vi "Autonomous Independent.vi"() -> ()   [LabVIEW 2016]
doc: "This VI is called when autonomous begins, and will automatically be terminated when autonomous ends. You can carry out timed or sensor driven robot movement independently without needing to return to the caller."
uses:
  <vilib>/Rock Robotics/WPI/ThirdParty/CanMotor/TalonSRX/WPI_CANTalonSRX_APIFeedbackSelect.ctl
  <vilib>/Rock Robotics/WPI/ThirdParty/CanMotor/TalonSRX/WPI_CANTalonSRX_Params.ctl
  <vilib>/Rock Robotics/WPI/ThirdParty/CanMotor/TalonSRX/WPI_CANTalonSRX_APIControlMode.ctl
  <vilib>/Rock Robotics/WPI/Utilities/WPI_GetSetVariantRefNum.vi
  <vilib>/Rock Robotics/Network Tables/NT Read String.vi
  <vilib>/Rock Robotics/Network Tables/NT Write Numeric Array.vi
  <vilib>/Rock Robotics/WPI/RobotDrive/WPI_RobotDriveArcadeDrive_Standard(NoSaturation).vi
  Robot Global Data.vi
panel:
  out "RIGHT SIDE":dbl
  out "Encoder Position 4":dbl
  out "Encoder Position 3":dbl
  out "Encoder Position":dbl
  out "Encoder Position 2":dbl
  # "Be sure to right-click and choose Data Operations>>Make Current Value default if you want to save the array values with the VI"
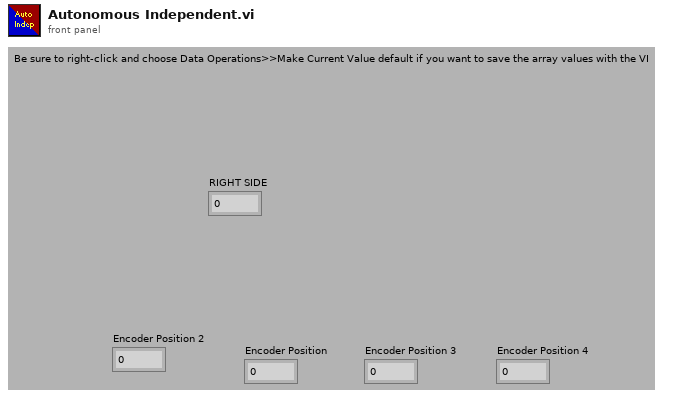
[diagram p1: front panel]
types:
  T1 = typedef "WPI_JoystickDevRef.ctl" = cluster{"Device":T2}
  T2 = typedef "WPI_JoystickDeviceEnum.ctl" = enum16{"USB 0", "USB 1", "USB 2", "USB 3", "USB 4", "USB 5"}
  T3 = typedef "WPI_EncoderDevRef.ctl" = cluster{"DevStatus":errorcluster, "EncoderIndex":T4, "CounterIndex":T5, "DistancePerCount":dbl, "Decoding Type":T6}
  T4 = typedef "FPGA_EncoderIdx.ctl" = enum8{"Enc 0", "Enc 1", "Enc 2", "Enc 3", "Enc 4", "Enc 5", "Enc 6", "Enc 7", "Invalid"}
  T5 = typedef "FPGA_CounterCtrSystemIndex.ctl" = enum8{"Ctr 0", "Ctr 1", "Ctr 2", "Ctr 3", "Ctr 4", "Ctr 5", "Ctr 6", "Ctr 7", "Invalid"}
  T6 = typedef "WPI_EncoderType.ctl" = enum16{"1x", "2x", "4x"}
  T7 = typedef "WPI_MotorControlDeviceRef.ctl" = cluster{"DeviceStatus":errorcluster, "Type":T8, "PWM":cluster{"PWM Channel":T9, "DeadBand":T10}, "CAN":cluster{"Device Number":u8, "SetOutput VI Ref":variant, "GetOutput VI Ref":variant, "Enable VI Ref":variant, "Disable VI Ref":variant, "Data":variant}, "Invert":bool}
  T8 = typedef "WPI_MotorControlType.ctl" = enum16{"PWM", "CAN"}
  T9 = typedef "FPGA_DIOPWMChannel.ctl" = enum8{"PWM 0", "PWM 1", "PWM 2", "PWM 3", "PWM 4", "PWM 5", "PWM 6", "PWM 7", "PWM 8", "PWM 9", "PWM MXP 0", "PWM MXP 1", "PWM MXP 2", "PWM MXP 3", "PWM MXP 4", "PWM MXP 5", "PWM MXP 6", "PWM MXP 7", "PWM MXP 8", "PWM MXP 9", "Invalid"}
  T10 = typedef "WPI_PWMDeadband.ctl" = cluster{"Name":string, "maxPositivePwm":i32, "minPositivePwm":i32, "centerPwm":i32, "maxNegativePwm":i32, "minNegativePwm":i32, "angularRange":u16}
  T11 = typedef "WPI_RobotDriveDevRef.ctl" = cluster{"DevStatus":errorcluster, "Motors[]":T7[], "Square Inputs":bool, "Max Output":dbl}
  T12 = typedef "WPI_CANTalonSRX_APIFeedbackSelect.ctl" = enum16{"Digital Quadrature Encoder", "Analog Potentiometer", "Analog Encoder", "Count on Quad-A (Rising-Edge)", "Count on Quad-A (Falling-Edge)", "CTR Magnetic Enc (Absolute)", "CTR Magnetic Enc (Relative)", "Pulse Width"}
  T13 = typedef "WPI_CANTalonSRX_APIControlMode.ctl" = enum8{"Percent VBus", "Speed", "Position", "Slave", "Unchanged / Invalid", "Voltage Compensation", "Current", "Motion Profile", "Motion Magic"}
  T14 = typedef "WPI_CANTalonSRX_Params.ctl" = u8
  T15 = typedef "WPI_CANTalonSRX_GlobalStatus.ctl" = cluster{"Applied Throttle":dbl, "Module Enabled":bool, "CAN Error":errorcluster, "Closed Loop Error":dbl, "Forward Limit Switch Closed":bool, "Reverse Limit Switch Closed":bool, "Sensor Position":dbl, "Sensor Velocity":dbl, "Current":dbl, "Sticky Fault - Over Temp":bool, "Sticky Fault - Under Voltage":bool, "Sticky Fault - Forward Limit":bool, "Sticky Fault - Reverse Limit":bool, "Sticky Fault - Forward Soft Limit":bool, "Sticky Fault - Reverse Soft Limit":bool, "Brake is Enabled":bool, "Encoder Position":dbl, "Encoder Velocity":dbl, "Encoder Index Count":dbl, "Encoder A Pin State":bool, "Encoder B Pin State":bool, "Encoder Index Pin State":bool, "Analog In":dbl, "Analog In Velocity":dbl, "Temperature (C)":dbl, "Battery Voltage":dbl, "Control 5 Is Supported":bool, "Current Profile Slot Select":dbl, "Pos Div 8":bool, "Vel Div 4":bool, "Pulse Width Position":i32, "Pulse Width Velocity":i32, "Pulse Width Rise To Rise (us)":i32, "Pulse Width Rise To Fall (us)":i32, "Mot Prof Active Is Under Run":bool, "Mot Prof Active Has Under Run":bool, "Mot Prof Active Is Last":bool, "Mot Prof Active Velocity Only":bool, "Mot Prof Active Is Valid":bool, "Mot Prof Buffer Is Full":bool, "Mot Prof Active Profile Slot Select":i32, "Mot Prof NextID":i32, "Mot Prof Count":i32, "Mot Prof Active Velocity":dbl, "Mot Prof Active Position":dbl, "Mot Prof Output Enable":i32, "UsageFrame":u32}
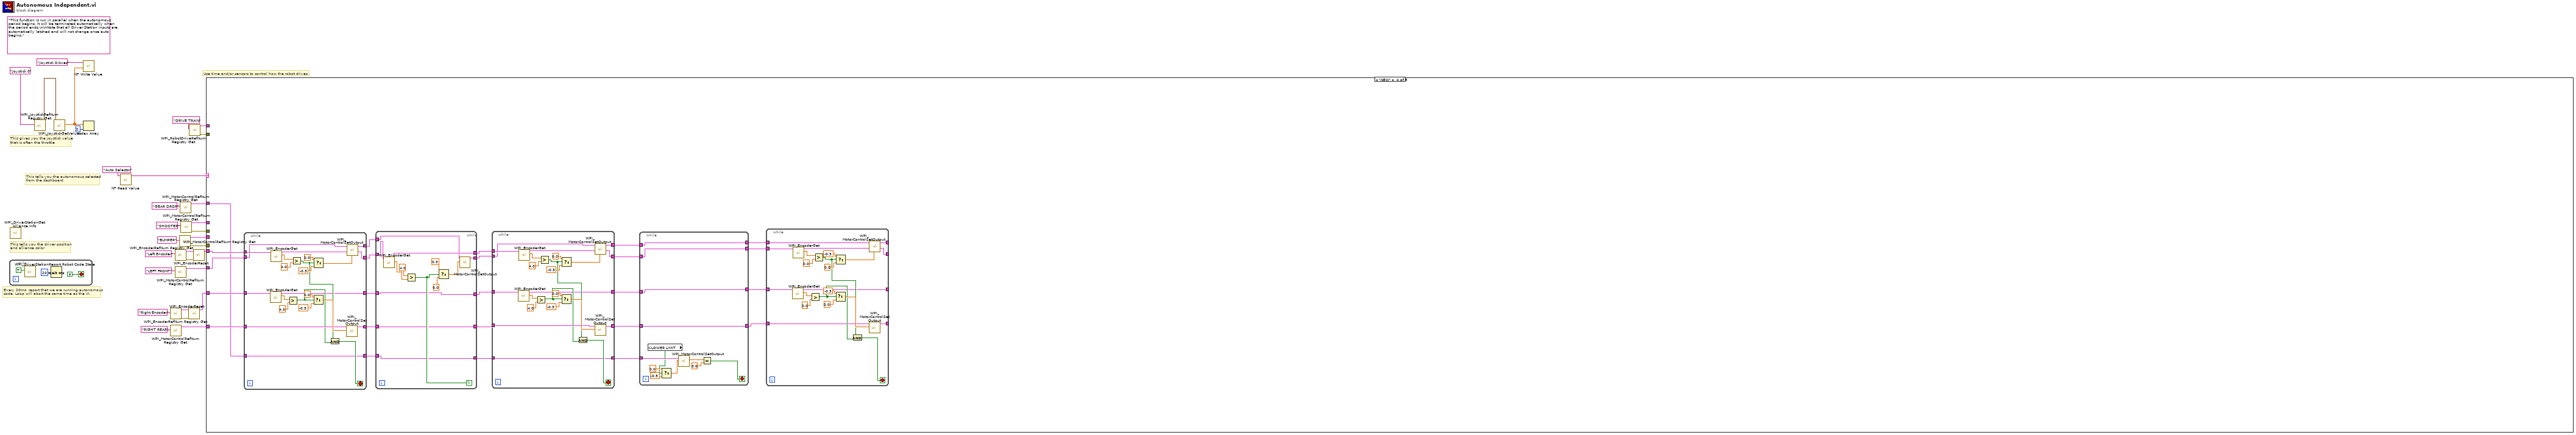
[diagram p0: block diagram]
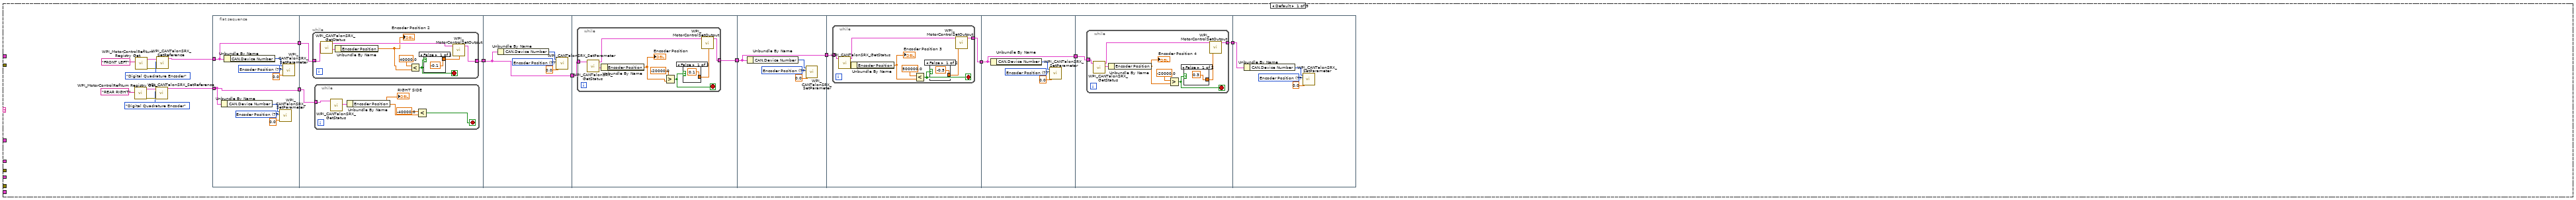
[diagram p2: hidden frame]
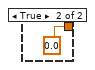
[diagram p3: hidden frame]
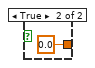
[diagram p4: hidden frame]
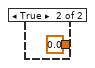
[diagram p5: hidden frame]
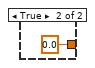
[diagram p6: hidden frame]
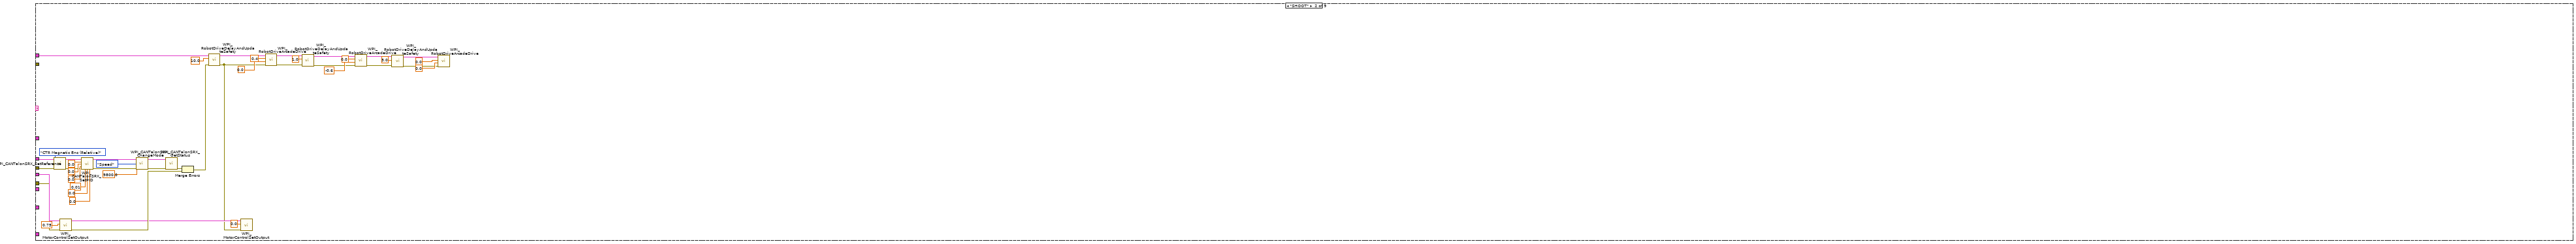
[diagram p7: hidden frame]
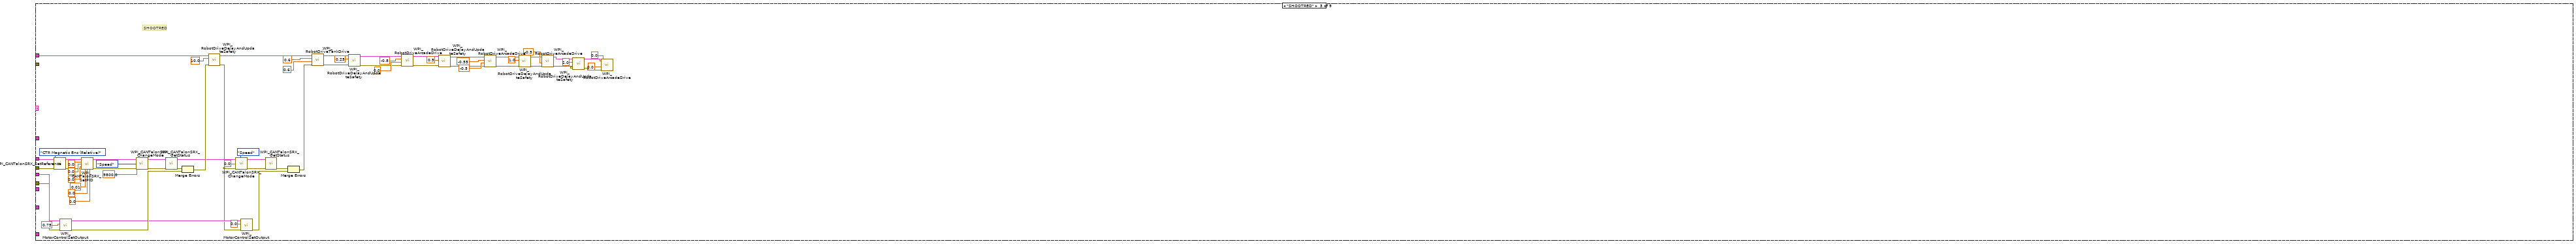
[diagram p8: hidden frame]
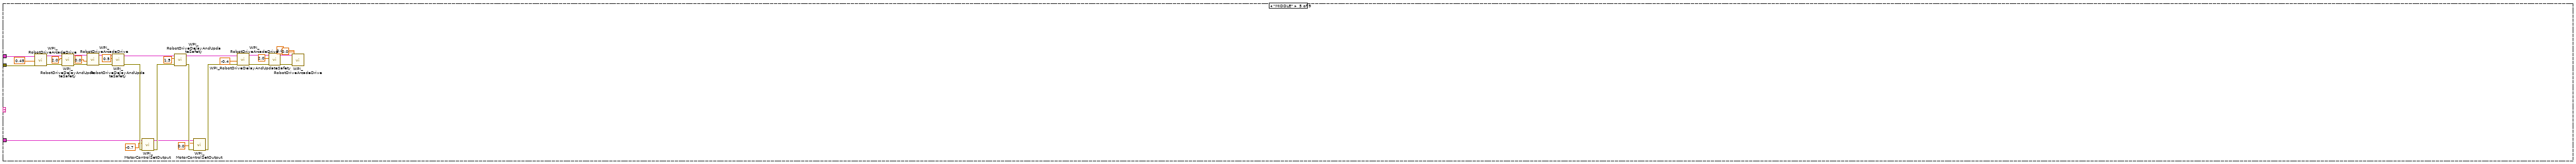
[diagram p9: hidden frame]
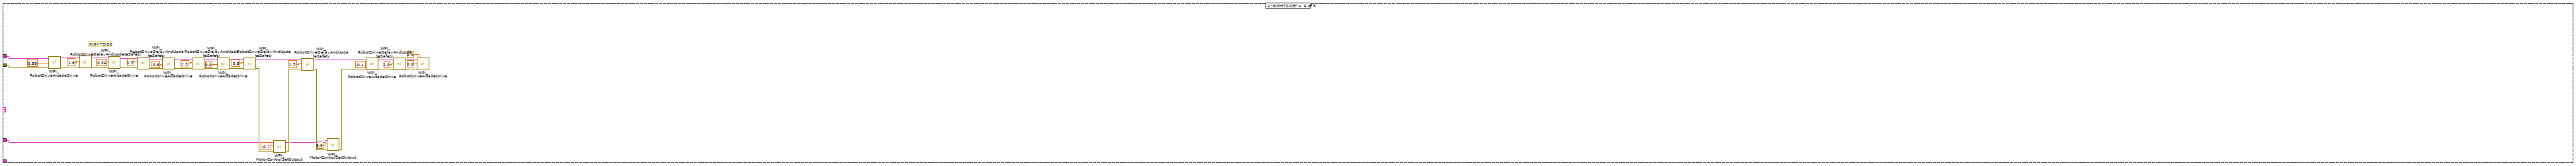
[diagram p10: hidden frame]
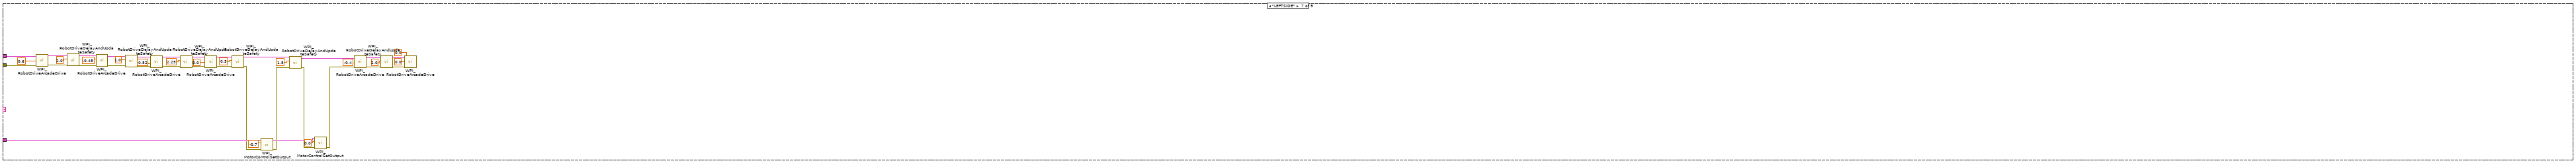
[diagram p11: hidden frame]
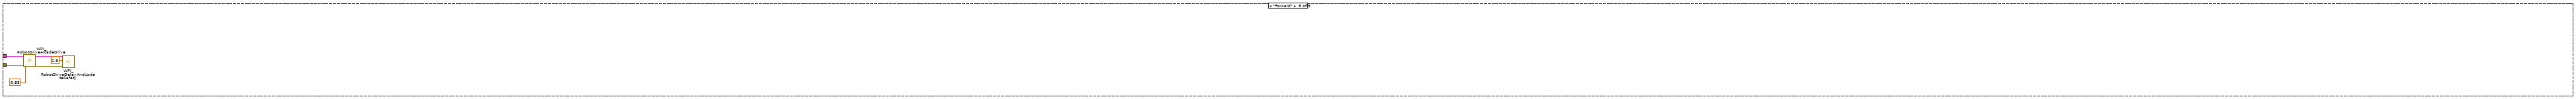
[diagram p12: hidden frame]
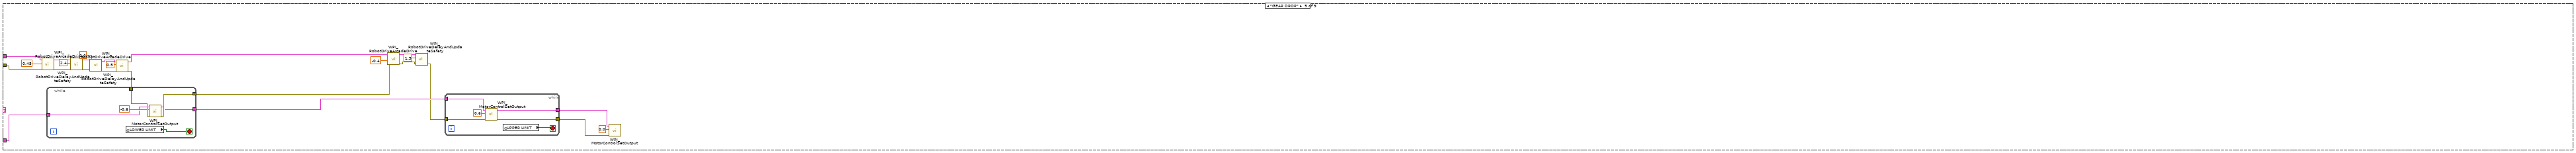
[diagram p13: hidden frame]
diagram:
  (unwired) "This function is run in parallel when the autonomous period begins. It will be terminated automatically when the period ends.\n\nNote that all Driver Station inputs are automatically latched and will not change once auto begins."
  # "Use time and/or sensors to control how the robot drives."
  # "This tells you the autonomous selected\nfrom the dashboard"
  # "Every 20ms, report that we are running autonomous\ncode. Loop will abort the same time as the VI."
  # "This gives you the joystick value\nthat is often the throttle"
  # "This tells you the driver position\nand alliance color"
  n1 = while {
    stop <- FALSE stop-if-true
    n2 = call <vilib>:"WPI_DriverStationReport Robot Code State.vi"("Autonomous"=TRUE) -> ()  [unwired: 10 in, 1 out]
    n3 = Wait (ms)(milliseconds to wait=u32 20) -> ()  [unwired: 1 out]
  }
  n4 = call <vilib>:"WPI_DriverStationGet Alliance Info.vi"() -> ()  [unwired: 12 out]
  n5 = call <vilib>:"WPI_JoystickRefNum Registry Get.vi"("refnum name"="Joystick 0") -> ("JoystickDevRef"=w29:T1)  [unwired: 1 in, 9 out]
  n6 = call <vilib>:"WPI_JoystickGetValues.vi"("JoystickDevRef"=w29) -> ("Axes"=w25:dbl[])  [unwired: 6 in, 4 out]
  n7 = call-poly <vilib>:"NT Write Value.vi"("Numeric Array"=w25, "Name"="Joystick 0/Axes") -> ()  [unwired: 9 in, 1 out]
  n8 = Index Array(array=w25, index=2) -> ()  [unwired: 1 out]
  n9 = call-poly <vilib>:"NT Read Value.vi"("Name"="Auto Selector") -> ("String"=w26:string)  [unwired: 9 in, 1 out]
  n10 = call <vilib>:"WPI_EncoderRefNum Registry Get.vi"("refnum name"="Right Encoder") -> ("error out"=w3:errorcluster, "EncoderDevRef"=w4:T3)  [unwired: 9 in]
  n11 = call <vilib>:"WPI_MotorControlRefNum Registry Get.vi"("refnum name"="RIGHT REAR") -> ("MotorControlDevRef"=w2:T7)  [unwired: 9 in, 1 out]
  n12 = call <vilib>:"WPI_EncoderRefNum Registry Get.vi"("refnum name"="Left Encoder") -> ("error out"=w12:errorcluster, "EncoderDevRef"=w11:T3)  [unwired: 9 in]
  n13 = call <vilib>:"WPI_MotorControlRefNum Registry Get.vi"("refnum name"="LEFT FRONT") -> ("MotorControlDevRef"=w7:T7)  [unwired: 9 in, 1 out]
  n14 = call <vilib>:"WPI_MotorControlRefNum Registry Get.vi"("refnum name"="BUMPER") -> ("error out"=w14:errorcluster, "MotorControlDevRef"=w15:T7)  [unwired: 9 in]
  n15 = call <vilib>:"WPI_MotorControlRefNum Registry Get.vi"("refnum name"="GEAR DROP") -> ("MotorControlDevRef"=w19:T7)  [unwired: 9 in, 1 out]
  n16 = call <vilib>:"WPI_MotorControlRefNum Registry Get.vi"("refnum name"="SHOOTER") -> ("error out"=w16:errorcluster, "MotorControlDevRef"=w17:T7)  [unwired: 9 in]
  n17 = call <vilib>:"WPI_EncoderReset.vi"("error in (no error)"=w3, "EncoderDevRef"=w4) -> ("EncoderDevRef"=w1:T3)  [unwired: 8 in, 1 out]
  n18 = call <vilib>:"WPI_RobotDriveRefNum Registry Get.vi"("refnum name"="DRIVE TRAIN") -> ("error out"=w21:errorcluster, "RobotDriveDevRef"=w22:T11)  [unwired: 9 in]
  n19 = call <vilib>:"WPI_EncoderReset.vi"("error in (no error)"=w12, "EncoderDevRef"=w11) -> ("EncoderDevRef"=w10:T3)  [unwired: 8 in, 1 out]
  n20 = case shown="\"NEW\"" w26 {
    tunnel: w22 -> [_ w157 w223 _ w386 w389 w472 w478 w503]
    tunnel: w21 -> [_ _ _ _ w385 w388 w471 w477 w502]
    tunnel: w19 -> [_ _ _ w249 w373 w387 w448 _ w483]
    tunnel: w17 -> [_ w163 w229 _ _ _ _ _ _]
    tunnel: w16 -> [_ w162 w228 _ _ _ _ _ _]
    tunnel: w15 -> [_ w148 w216 _ _ _ _ _ _]
    tunnel: w14 -> [_ w147 w215 _ _ _ _ _ _]
    tunnel: w10 -> [_ _ _ w263 _ _ _ _ _]
    tunnel: w7 -> [_ _ _ w262 _ _ _ _ _]
    tunnel: w2 -> [_ _ _ w260 _ _ _ _ _]
    tunnel: w1 -> [_ _ _ w261 _ _ _ _ _]
    frame Default {
      n21 = call <vilib>:"WPI_MotorControlRefNum Registry Get.vi"("refnum name"="REAR RIGHT") -> ("error out"=w38:errorcluster, "MotorControlDevRef"=w37:T7)  [unwired: 9 in]
      n22 = call <vilib>:"WPI_MotorControlRefNum Registry Get.vi"("refnum name"="FRONT LEFT") -> ("error out"=w50:errorcluster, "MotorControlDevRef"=w51:T7)  [unwired: 9 in]
      n23 = call <vilib>:"WPI_CANTalonSRX_SetReference.vi"("error in (no error)"=w38, "Feedback Reference"=WPI_CANTalonSRX_APIFeedbackSelect."Digital Quadrature Encoder", "CAN Talon SRX Ref"=w37) -> ("CAN Talon SRX Ref"=w35:T7)  [unwired: 7 in, 1 out]
      n24 = call <vilib>:"WPI_CANTalonSRX_SetReference.vi"("error in (no error)"=w50, "Feedback Reference"=WPI_CANTalonSRX_APIFeedbackSelect."Digital Quadrature Encoder", "CAN Talon SRX Ref"=w51) -> ("CAN Talon SRX Ref"=w46:T7)  [unwired: 7 in, 1 out]
      n25 = flat-sequence {
        tunnel: w46 -> [w57]
        tunnel: [w57] -> w45
        tunnel: w35 -> [w53]
        tunnel: [w53] -> w34
        tunnel: [w62] -> w48
        tunnel: w45 -> [w63]
        tunnel: w34 -> [w61]
        tunnel: w48 -> [w79]
        tunnel: [w79] -> w47
        tunnel: w47 -> [w84]
        tunnel: [w83] -> w44
        tunnel: w44 -> [w95]
        tunnel: [w95] -> w43
        tunnel: w43 -> [w100]
        tunnel: [w99] -> w42
        tunnel: w42 -> [w111]
        tunnel: [w111] -> w41
        tunnel: w41 -> [w116]
        tunnel: [w115] -> w40
        tunnel: w40 -> [w127]
        frame #0 {
          w55 = T14 77 items=["Slot 0 - P"=1, "Slot 0 - I"=2, "Slot 0 - D"=3, "Slot 0 - F"=4, "Slot 0 - I Zone"=5, "Slot 0 - Ramp Rate"=6, "Slot 1 - P"=11, "Slot 1 - I"=12, "Slot 1 - D"=13, "Slot 1 - F"=14, "Slot 1 - I Zone"=15, "Slot 1 - Ramp Rate"=16, "Soft Limit - Forward"=21, "Soft Limit - Reverse"=22, "Soft Limit - Forward Enable"=23, "Soft Limit - Reverse Enable"=24, "On Boot - Brake Mode"=31, "On Boot - Limit Normally Closed - Forward"=32, "On Boot - Limit Normally Closed - Reverse"=33, "On Boot - Limit Disabled - Forward"=34, "On Boot - Limit Disabled - Reverse"=35, "Fault - Over Temp"=41, "Fault - Under Voltage"=42, "Fault - Forward Limit"=43, "Fault - Reverse Limit"=44, "Fault - Hardware Failure"=45, "Fault - Forward Soft Limit"=46, "Fault - Reverse Soft Limit"=47, "Sticky Fault - Over Temp"=48, "Sticky Fault - Under Voltage"=49, "Sticky Fault - Forward Limit"=50, "Sticky Fault - Reverse Limit"=51, "Sticky Fault - Forward Soft Limit"=52, "Sticky Fault - Reverse Soft Limit"=53, "Applied Throttle"=61, "Closed-Loop Error"=62, "Select Feedback Device"=63, "Reverse Closed-Loop Output"=64, "Mode Select"=65, "Profile Slot Select"=66, "Ramp Throttle"=67, "Reverse Feedback Sensor"=68, "Limit Switch Enabled"=69, "Limit Switch Closed - Forward"=70, "Limit Switch Closed - Reverse"=71, "Sensor Position"=73, "Sensor Velocity"=74, "Current"=75, "Brake is Enabled"=76, "Encoder Position"=77, "Encoder Velocity"=78, "Encoder Index Rise Events"=79, "Encoder A Pin State"=80, "Encoder B Pin State"=81, "Encoder Index Pin State"=82, "Analog In with Overflow"=83, "Analog In Velocity"=84, "Temperature"=85, "Battery Voltage"=86, "Reset Count"=87, "Reset Flags"=88, "Firmware Version"=89, "Settings Changed"=90, "Quad Filter Enable"=91, "Ignore Disable Broadcast"=92, "I Accumulator"=93, "Status 1 Frame Rate Ms"=94, "Status 2 Frame Rate Ms"=95, "Status 3 Frame Rate Ms"=96, "Status 4 Frame Rate Ms"=97, "Status 6 Frame Rate Ms"=98, "Status 7 Frame Rate Ms"=99, "Enable Index Pin Clear Position"=100, "Peak Positive Output"=104, "Nominal Positive Output"=105, "Peak Negative Output"=106, "Nominal Negative Output"=107, "Quad Index Pin Polarity"=108, "Status 8 Frame Rate Ms"=109, "Allow Position Overflow"=110, "Slot 0 - Allowable Closed-Loop Error"=111, "Number Potentiometer Turns"=112, "Encoder Codes Per Rev"=113, "Pulse Width Decoded Position"=114, "Analog Position"=115, "Voltage Compensation Rate (V/s)"=116, "Slot 1 - Allowable Closed-Loop Error"=117, "Motion Profile Has Underrun Err"=119, "Reserved 120"=120, "Legacy Control Mode"=121, "Motion Magic Acceleration"=122, "Motion Magic Cruise Velocity"=123, "Status 10 Frame Rate"=124, "Current Limit Threshold"=125, "CustomParam0"=137, "CustomParam1"=138, "PersStorageSaving"=139, "ClearPositionOnLimitF"=144, "ClearPositionOnLimitR"=145, "NominalBatteryVoltage"=146, "SampleVelocityPeriod"=147, "SampleVelocityWindow"=148] ("Parameter")
          w59 = T14 77 items=["Slot 0 - P"=1, "Slot 0 - I"=2, "Slot 0 - D"=3, "Slot 0 - F"=4, "Slot 0 - I Zone"=5, "Slot 0 - Ramp Rate"=6, "Slot 1 - P"=11, "Slot 1 - I"=12, "Slot 1 - D"=13, "Slot 1 - F"=14, "Slot 1 - I Zone"=15, "Slot 1 - Ramp Rate"=16, "Soft Limit - Forward"=21, "Soft Limit - Reverse"=22, "Soft Limit - Forward Enable"=23, "Soft Limit - Reverse Enable"=24, "On Boot - Brake Mode"=31, "On Boot - Limit Normally Closed - Forward"=32, "On Boot - Limit Normally Closed - Reverse"=33, "On Boot - Limit Disabled - Forward"=34, "On Boot - Limit Disabled - Reverse"=35, "Fault - Over Temp"=41, "Fault - Under Voltage"=42, "Fault - Forward Limit"=43, "Fault - Reverse Limit"=44, "Fault - Hardware Failure"=45, "Fault - Forward Soft Limit"=46, "Fault - Reverse Soft Limit"=47, "Sticky Fault - Over Temp"=48, "Sticky Fault - Under Voltage"=49, "Sticky Fault - Forward Limit"=50, "Sticky Fault - Reverse Limit"=51, "Sticky Fault - Forward Soft Limit"=52, "Sticky Fault - Reverse Soft Limit"=53, "Applied Throttle"=61, "Closed-Loop Error"=62, "Select Feedback Device"=63, "Reverse Closed-Loop Output"=64, "Mode Select"=65, "Profile Slot Select"=66, "Ramp Throttle"=67, "Reverse Feedback Sensor"=68, "Limit Switch Enabled"=69, "Limit Switch Closed - Forward"=70, "Limit Switch Closed - Reverse"=71, "Sensor Position"=73, "Sensor Velocity"=74, "Current"=75, "Brake is Enabled"=76, "Encoder Position"=77, "Encoder Velocity"=78, "Encoder Index Rise Events"=79, "Encoder A Pin State"=80, "Encoder B Pin State"=81, "Encoder Index Pin State"=82, "Analog In with Overflow"=83, "Analog In Velocity"=84, "Temperature"=85, "Battery Voltage"=86, "Reset Count"=87, "Reset Flags"=88, "Firmware Version"=89, "Settings Changed"=90, "Quad Filter Enable"=91, "Ignore Disable Broadcast"=92, "I Accumulator"=93, "Status 1 Frame Rate Ms"=94, "Status 2 Frame Rate Ms"=95, "Status 3 Frame Rate Ms"=96, "Status 4 Frame Rate Ms"=97, "Status 6 Frame Rate Ms"=98, "Status 7 Frame Rate Ms"=99, "Enable Index Pin Clear Position"=100, "Peak Positive Output"=104, "Nominal Positive Output"=105, "Peak Negative Output"=106, "Nominal Negative Output"=107, "Quad Index Pin Polarity"=108, "Status 8 Frame Rate Ms"=109, "Allow Position Overflow"=110, "Slot 0 - Allowable Closed-Loop Error"=111, "Number Potentiometer Turns"=112, "Encoder Codes Per Rev"=113, "Pulse Width Decoded Position"=114, "Analog Position"=115, "Voltage Compensation Rate (V/s)"=116, "Slot 1 - Allowable Closed-Loop Error"=117, "Motion Profile Has Underrun Err"=119, "Reserved 120"=120, "Legacy Control Mode"=121, "Motion Magic Acceleration"=122, "Motion Magic Cruise Velocity"=123, "Status 10 Frame Rate"=124, "Current Limit Threshold"=125, "CustomParam0"=137, "CustomParam1"=138, "PersStorageSaving"=139, "ClearPositionOnLimitF"=144, "ClearPositionOnLimitR"=145, "NominalBatteryVoltage"=146, "SampleVelocityPeriod"=147, "SampleVelocityWindow"=148] ("Parameter")
          n26 = Unbundle By Name(w53) -> ("CAN.Device Number"=w54:u8)
          n27 = Unbundle By Name(w57) -> ("CAN.Device Number"=w60:u8)
          n28 = call <vilib>:"WPI_CANTalonSRX_SetParameter.vi"("Value"=0.0, "Parameter"=w55, "Device ID (0)"=w54) -> ()  [unwired: 7 in, 2 out]
          n29 = call <vilib>:"WPI_CANTalonSRX_SetParameter.vi"("Value"=0.0, "Parameter"=w59, "Device ID (0)"=w60) -> ()  [unwired: 7 in, 2 out]
        }
        frame #1 {
          n30 = while {
            tunnel: w63 -> [w70]
            tunnel: [w69] -> w62
            stop <- w73 stop-if-true
            n31 = call <vilib>:"WPI_CANTalonSRX_GetStatus.vi"("CAN Talon SRX Ref"=w70) -> ("Talon SRX Status"=w76:T15, "CAN Talon SRX Ref"=w75:T7)  [unwired: 8 in, 1 out]
            n32 = Unbundle By Name(w76) -> ("Encoder Position"=w72:dbl)
            "Encoder Position 2" <- w72
            n33 = Less?(x=40000.0, y=w72) -> (x < y?=w73:bool)
            n34 = case shown="False" w73 {
              tunnel: [-0.1 ("x") 0.0 ("x")] -> w74
              frame False {
              }
              frame True {
              }
            }
            n35 = call <vilib>:"WPI_MotorControlSetOutput.vi"("Output"=w74, "MotorControlDevRef"=w75) -> ("MotorControlDevRef"=w69:T7)  [unwired: 7 in, 2 out]
          }
          n36 = while {
            tunnel: w61 -> [w68]
            stop <- w65 stop-if-true
            n37 = call <vilib>:"WPI_CANTalonSRX_GetStatus.vi"("CAN Talon SRX Ref"=w68) -> ("Talon SRX Status"=w64:T15)  [unwired: 8 in, 2 out]
            n38 = Unbundle By Name(w64) -> ("Encoder Position"=w67:dbl)
            "RIGHT SIDE" <- w67
            n39 = Less?(x=-40000.0, y=w67) -> (x < y?=w65:bool)
          }
        }
        frame #2 {
          w81 = T14 77 items=["Slot 0 - P"=1, "Slot 0 - I"=2, "Slot 0 - D"=3, "Slot 0 - F"=4, "Slot 0 - I Zone"=5, "Slot 0 - Ramp Rate"=6, "Slot 1 - P"=11, "Slot 1 - I"=12, "Slot 1 - D"=13, "Slot 1 - F"=14, "Slot 1 - I Zone"=15, "Slot 1 - Ramp Rate"=16, "Soft Limit - Forward"=21, "Soft Limit - Reverse"=22, "Soft Limit - Forward Enable"=23, "Soft Limit - Reverse Enable"=24, "On Boot - Brake Mode"=31, "On Boot - Limit Normally Closed - Forward"=32, "On Boot - Limit Normally Closed - Reverse"=33, "On Boot - Limit Disabled - Forward"=34, "On Boot - Limit Disabled - Reverse"=35, "Fault - Over Temp"=41, "Fault - Under Voltage"=42, "Fault - Forward Limit"=43, "Fault - Reverse Limit"=44, "Fault - Hardware Failure"=45, "Fault - Forward Soft Limit"=46, "Fault - Reverse Soft Limit"=47, "Sticky Fault - Over Temp"=48, "Sticky Fault - Under Voltage"=49, "Sticky Fault - Forward Limit"=50, "Sticky Fault - Reverse Limit"=51, "Sticky Fault - Forward Soft Limit"=52, "Sticky Fault - Reverse Soft Limit"=53, "Applied Throttle"=61, "Closed-Loop Error"=62, "Select Feedback Device"=63, "Reverse Closed-Loop Output"=64, "Mode Select"=65, "Profile Slot Select"=66, "Ramp Throttle"=67, "Reverse Feedback Sensor"=68, "Limit Switch Enabled"=69, "Limit Switch Closed - Forward"=70, "Limit Switch Closed - Reverse"=71, "Sensor Position"=73, "Sensor Velocity"=74, "Current"=75, "Brake is Enabled"=76, "Encoder Position"=77, "Encoder Velocity"=78, "Encoder Index Rise Events"=79, "Encoder A Pin State"=80, "Encoder B Pin State"=81, "Encoder Index Pin State"=82, "Analog In with Overflow"=83, "Analog In Velocity"=84, "Temperature"=85, "Battery Voltage"=86, "Reset Count"=87, "Reset Flags"=88, "Firmware Version"=89, "Settings Changed"=90, "Quad Filter Enable"=91, "Ignore Disable Broadcast"=92, "I Accumulator"=93, "Status 1 Frame Rate Ms"=94, "Status 2 Frame Rate Ms"=95, "Status 3 Frame Rate Ms"=96, "Status 4 Frame Rate Ms"=97, "Status 6 Frame Rate Ms"=98, "Status 7 Frame Rate Ms"=99, "Enable Index Pin Clear Position"=100, "Peak Positive Output"=104, "Nominal Positive Output"=105, "Peak Negative Output"=106, "Nominal Negative Output"=107, "Quad Index Pin Polarity"=108, "Status 8 Frame Rate Ms"=109, "Allow Position Overflow"=110, "Slot 0 - Allowable Closed-Loop Error"=111, "Number Potentiometer Turns"=112, "Encoder Codes Per Rev"=113, "Pulse Width Decoded Position"=114, "Analog Position"=115, "Voltage Compensation Rate (V/s)"=116, "Slot 1 - Allowable Closed-Loop Error"=117, "Motion Profile Has Underrun Err"=119, "Reserved 120"=120, "Legacy Control Mode"=121, "Motion Magic Acceleration"=122, "Motion Magic Cruise Velocity"=123, "Status 10 Frame Rate"=124, "Current Limit Threshold"=125, "CustomParam0"=137, "CustomParam1"=138, "PersStorageSaving"=139, "ClearPositionOnLimitF"=144, "ClearPositionOnLimitR"=145, "NominalBatteryVoltage"=146, "SampleVelocityPeriod"=147, "SampleVelocityWindow"=148] ("Parameter")
          n40 = Unbundle By Name(w79) -> ("CAN.Device Number"=w82:u8)
          n41 = call <vilib>:"WPI_CANTalonSRX_SetParameter.vi"("Value"=0.0, "Parameter"=w81, "Device ID (0)"=w82) -> ()  [unwired: 7 in, 2 out]
        }
        frame #3 {
          n42 = while {
            tunnel: w84 -> [w86]
            tunnel: [w85] -> w83
            stop <- w89 stop-if-true
            n43 = call <vilib>:"WPI_CANTalonSRX_GetStatus.vi"("CAN Talon SRX Ref"=w86) -> ("Talon SRX Status"=w92:T15, "CAN Talon SRX Ref"=w91:T7)  [unwired: 8 in, 1 out]
            n44 = Unbundle By Name(w92) -> ("Encoder Position"=w88:dbl)
            "Encoder Position" <- w88
            n45 = Greater?(x=-20000.0 ("y"), y=w88) -> (0:w89:bool)
            n46 = case shown="False" w89 {
              tunnel: [0.1 ("x") 0.0 ("x")] -> w90
              frame False {
              }
              frame True {
              }
            }
            n47 = call <vilib>:"WPI_MotorControlSetOutput.vi"("Output"=w90, "MotorControlDevRef"=w91) -> ("MotorControlDevRef"=w85:T7)  [unwired: 7 in, 2 out]
          }
        }
        frame #4 {
          w97 = T14 77 items=["Slot 0 - P"=1, "Slot 0 - I"=2, "Slot 0 - D"=3, "Slot 0 - F"=4, "Slot 0 - I Zone"=5, "Slot 0 - Ramp Rate"=6, "Slot 1 - P"=11, "Slot 1 - I"=12, "Slot 1 - D"=13, "Slot 1 - F"=14, "Slot 1 - I Zone"=15, "Slot 1 - Ramp Rate"=16, "Soft Limit - Forward"=21, "Soft Limit - Reverse"=22, "Soft Limit - Forward Enable"=23, "Soft Limit - Reverse Enable"=24, "On Boot - Brake Mode"=31, "On Boot - Limit Normally Closed - Forward"=32, "On Boot - Limit Normally Closed - Reverse"=33, "On Boot - Limit Disabled - Forward"=34, "On Boot - Limit Disabled - Reverse"=35, "Fault - Over Temp"=41, "Fault - Under Voltage"=42, "Fault - Forward Limit"=43, "Fault - Reverse Limit"=44, "Fault - Hardware Failure"=45, "Fault - Forward Soft Limit"=46, "Fault - Reverse Soft Limit"=47, "Sticky Fault - Over Temp"=48, "Sticky Fault - Under Voltage"=49, "Sticky Fault - Forward Limit"=50, "Sticky Fault - Reverse Limit"=51, "Sticky Fault - Forward Soft Limit"=52, "Sticky Fault - Reverse Soft Limit"=53, "Applied Throttle"=61, "Closed-Loop Error"=62, "Select Feedback Device"=63, "Reverse Closed-Loop Output"=64, "Mode Select"=65, "Profile Slot Select"=66, "Ramp Throttle"=67, "Reverse Feedback Sensor"=68, "Limit Switch Enabled"=69, "Limit Switch Closed - Forward"=70, "Limit Switch Closed - Reverse"=71, "Sensor Position"=73, "Sensor Velocity"=74, "Current"=75, "Brake is Enabled"=76, "Encoder Position"=77, "Encoder Velocity"=78, "Encoder Index Rise Events"=79, "Encoder A Pin State"=80, "Encoder B Pin State"=81, "Encoder Index Pin State"=82, "Analog In with Overflow"=83, "Analog In Velocity"=84, "Temperature"=85, "Battery Voltage"=86, "Reset Count"=87, "Reset Flags"=88, "Firmware Version"=89, "Settings Changed"=90, "Quad Filter Enable"=91, "Ignore Disable Broadcast"=92, "I Accumulator"=93, "Status 1 Frame Rate Ms"=94, "Status 2 Frame Rate Ms"=95, "Status 3 Frame Rate Ms"=96, "Status 4 Frame Rate Ms"=97, "Status 6 Frame Rate Ms"=98, "Status 7 Frame Rate Ms"=99, "Enable Index Pin Clear Position"=100, "Peak Positive Output"=104, "Nominal Positive Output"=105, "Peak Negative Output"=106, "Nominal Negative Output"=107, "Quad Index Pin Polarity"=108, "Status 8 Frame Rate Ms"=109, "Allow Position Overflow"=110, "Slot 0 - Allowable Closed-Loop Error"=111, "Number Potentiometer Turns"=112, "Encoder Codes Per Rev"=113, "Pulse Width Decoded Position"=114, "Analog Position"=115, "Voltage Compensation Rate (V/s)"=116, "Slot 1 - Allowable Closed-Loop Error"=117, "Motion Profile Has Underrun Err"=119, "Reserved 120"=120, "Legacy Control Mode"=121, "Motion Magic Acceleration"=122, "Motion Magic Cruise Velocity"=123, "Status 10 Frame Rate"=124, "Current Limit Threshold"=125, "CustomParam0"=137, "CustomParam1"=138, "PersStorageSaving"=139, "ClearPositionOnLimitF"=144, "ClearPositionOnLimitR"=145, "NominalBatteryVoltage"=146, "SampleVelocityPeriod"=147, "SampleVelocityWindow"=148] ("Parameter")
          n48 = Unbundle By Name(w95) -> ("CAN.Device Number"=w98:u8)
          n49 = call <vilib>:"WPI_CANTalonSRX_SetParameter.vi"("Value"=0.0, "Parameter"=w97, "Device ID (0)"=w98) -> ()  [unwired: 7 in, 2 out]
        }
        frame #5 {
          n50 = while {
            tunnel: w100 -> [w102]
            tunnel: [w101] -> w99
            stop <- w105 stop-if-true
            n51 = call <vilib>:"WPI_CANTalonSRX_GetStatus.vi"("CAN Talon SRX Ref"=w102) -> ("Talon SRX Status"=w108:T15, "CAN Talon SRX Ref"=w107:T7)  [unwired: 8 in, 1 out]
            n52 = Unbundle By Name(w108) -> ("Encoder Position"=w104:dbl)
            "Encoder Position 3" <- w104
            n53 = Less?(x=500000.0, y=w104) -> (x < y?=w105:bool)
            n54 = case shown="False" w105 {
              tunnel: [-0.5 ("x") 0.0 ("x")] -> w106
              frame False {
              }
              frame True {
              }
            }
            n55 = call <vilib>:"WPI_MotorControlSetOutput.vi"("Output"=w106, "MotorControlDevRef"=w107) -> ("MotorControlDevRef"=w101:T7)  [unwired: 7 in, 2 out]
          }
        }
        frame #6 {
          w113 = T14 77 items=["Slot 0 - P"=1, "Slot 0 - I"=2, "Slot 0 - D"=3, "Slot 0 - F"=4, "Slot 0 - I Zone"=5, "Slot 0 - Ramp Rate"=6, "Slot 1 - P"=11, "Slot 1 - I"=12, "Slot 1 - D"=13, "Slot 1 - F"=14, "Slot 1 - I Zone"=15, "Slot 1 - Ramp Rate"=16, "Soft Limit - Forward"=21, "Soft Limit - Reverse"=22, "Soft Limit - Forward Enable"=23, "Soft Limit - Reverse Enable"=24, "On Boot - Brake Mode"=31, "On Boot - Limit Normally Closed - Forward"=32, "On Boot - Limit Normally Closed - Reverse"=33, "On Boot - Limit Disabled - Forward"=34, "On Boot - Limit Disabled - Reverse"=35, "Fault - Over Temp"=41, "Fault - Under Voltage"=42, "Fault - Forward Limit"=43, "Fault - Reverse Limit"=44, "Fault - Hardware Failure"=45, "Fault - Forward Soft Limit"=46, "Fault - Reverse Soft Limit"=47, "Sticky Fault - Over Temp"=48, "Sticky Fault - Under Voltage"=49, "Sticky Fault - Forward Limit"=50, "Sticky Fault - Reverse Limit"=51, "Sticky Fault - Forward Soft Limit"=52, "Sticky Fault - Reverse Soft Limit"=53, "Applied Throttle"=61, "Closed-Loop Error"=62, "Select Feedback Device"=63, "Reverse Closed-Loop Output"=64, "Mode Select"=65, "Profile Slot Select"=66, "Ramp Throttle"=67, "Reverse Feedback Sensor"=68, "Limit Switch Enabled"=69, "Limit Switch Closed - Forward"=70, "Limit Switch Closed - Reverse"=71, "Sensor Position"=73, "Sensor Velocity"=74, "Current"=75, "Brake is Enabled"=76, "Encoder Position"=77, "Encoder Velocity"=78, "Encoder Index Rise Events"=79, "Encoder A Pin State"=80, "Encoder B Pin State"=81, "Encoder Index Pin State"=82, "Analog In with Overflow"=83, "Analog In Velocity"=84, "Temperature"=85, "Battery Voltage"=86, "Reset Count"=87, "Reset Flags"=88, "Firmware Version"=89, "Settings Changed"=90, "Quad Filter Enable"=91, "Ignore Disable Broadcast"=92, "I Accumulator"=93, "Status 1 Frame Rate Ms"=94, "Status 2 Frame Rate Ms"=95, "Status 3 Frame Rate Ms"=96, "Status 4 Frame Rate Ms"=97, "Status 6 Frame Rate Ms"=98, "Status 7 Frame Rate Ms"=99, "Enable Index Pin Clear Position"=100, "Peak Positive Output"=104, "Nominal Positive Output"=105, "Peak Negative Output"=106, "Nominal Negative Output"=107, "Quad Index Pin Polarity"=108, "Status 8 Frame Rate Ms"=109, "Allow Position Overflow"=110, "Slot 0 - Allowable Closed-Loop Error"=111, "Number Potentiometer Turns"=112, "Encoder Codes Per Rev"=113, "Pulse Width Decoded Position"=114, "Analog Position"=115, "Voltage Compensation Rate (V/s)"=116, "Slot 1 - Allowable Closed-Loop Error"=117, "Motion Profile Has Underrun Err"=119, "Reserved 120"=120, "Legacy Control Mode"=121, "Motion Magic Acceleration"=122, "Motion Magic Cruise Velocity"=123, "Status 10 Frame Rate"=124, "Current Limit Threshold"=125, "CustomParam0"=137, "CustomParam1"=138, "PersStorageSaving"=139, "ClearPositionOnLimitF"=144, "ClearPositionOnLimitR"=145, "NominalBatteryVoltage"=146, "SampleVelocityPeriod"=147, "SampleVelocityWindow"=148] ("Parameter")
          n56 = Unbundle By Name(w111) -> ("CAN.Device Number"=w112:u8)
          n57 = call <vilib>:"WPI_CANTalonSRX_SetParameter.vi"("Value"=0.0, "Parameter"=w113, "Device ID (0)"=w112) -> ()  [unwired: 7 in, 2 out]
        }
        frame #7 {
          n58 = while {
            tunnel: w116 -> [w118]
            tunnel: [w117] -> w115
            stop <- w121 stop-if-true
            n59 = call <vilib>:"WPI_CANTalonSRX_GetStatus.vi"("CAN Talon SRX Ref"=w118) -> ("Talon SRX Status"=w124:T15, "CAN Talon SRX Ref"=w123:T7)  [unwired: 8 in, 1 out]
            n60 = Unbundle By Name(w124) -> ("Encoder Position"=w120:dbl)
            "Encoder Position 4" <- w120
            n61 = Greater?(x=-20000.0, y=w120) -> (0:w121:bool)
            n62 = case shown="False" w121 {
              tunnel: [0.3 ("x") 0.0 ("x")] -> w122
              frame False {
              }
              frame True {
              }
            }
            n63 = call <vilib>:"WPI_MotorControlSetOutput.vi"("Output"=w122, "MotorControlDevRef"=w123) -> ("MotorControlDevRef"=w117:T7)  [unwired: 7 in, 2 out]
          }
        }
        frame #8 {
          w129 = T14 77 items=["Slot 0 - P"=1, "Slot 0 - I"=2, "Slot 0 - D"=3, "Slot 0 - F"=4, "Slot 0 - I Zone"=5, "Slot 0 - Ramp Rate"=6, "Slot 1 - P"=11, "Slot 1 - I"=12, "Slot 1 - D"=13, "Slot 1 - F"=14, "Slot 1 - I Zone"=15, "Slot 1 - Ramp Rate"=16, "Soft Limit - Forward"=21, "Soft Limit - Reverse"=22, "Soft Limit - Forward Enable"=23, "Soft Limit - Reverse Enable"=24, "On Boot - Brake Mode"=31, "On Boot - Limit Normally Closed - Forward"=32, "On Boot - Limit Normally Closed - Reverse"=33, "On Boot - Limit Disabled - Forward"=34, "On Boot - Limit Disabled - Reverse"=35, "Fault - Over Temp"=41, "Fault - Under Voltage"=42, "Fault - Forward Limit"=43, "Fault - Reverse Limit"=44, "Fault - Hardware Failure"=45, "Fault - Forward Soft Limit"=46, "Fault - Reverse Soft Limit"=47, "Sticky Fault - Over Temp"=48, "Sticky Fault - Under Voltage"=49, "Sticky Fault - Forward Limit"=50, "Sticky Fault - Reverse Limit"=51, "Sticky Fault - Forward Soft Limit"=52, "Sticky Fault - Reverse Soft Limit"=53, "Applied Throttle"=61, "Closed-Loop Error"=62, "Select Feedback Device"=63, "Reverse Closed-Loop Output"=64, "Mode Select"=65, "Profile Slot Select"=66, "Ramp Throttle"=67, "Reverse Feedback Sensor"=68, "Limit Switch Enabled"=69, "Limit Switch Closed - Forward"=70, "Limit Switch Closed - Reverse"=71, "Sensor Position"=73, "Sensor Velocity"=74, "Current"=75, "Brake is Enabled"=76, "Encoder Position"=77, "Encoder Velocity"=78, "Encoder Index Rise Events"=79, "Encoder A Pin State"=80, "Encoder B Pin State"=81, "Encoder Index Pin State"=82, "Analog In with Overflow"=83, "Analog In Velocity"=84, "Temperature"=85, "Battery Voltage"=86, "Reset Count"=87, "Reset Flags"=88, "Firmware Version"=89, "Settings Changed"=90, "Quad Filter Enable"=91, "Ignore Disable Broadcast"=92, "I Accumulator"=93, "Status 1 Frame Rate Ms"=94, "Status 2 Frame Rate Ms"=95, "Status 3 Frame Rate Ms"=96, "Status 4 Frame Rate Ms"=97, "Status 6 Frame Rate Ms"=98, "Status 7 Frame Rate Ms"=99, "Enable Index Pin Clear Position"=100, "Peak Positive Output"=104, "Nominal Positive Output"=105, "Peak Negative Output"=106, "Nominal Negative Output"=107, "Quad Index Pin Polarity"=108, "Status 8 Frame Rate Ms"=109, "Allow Position Overflow"=110, "Slot 0 - Allowable Closed-Loop Error"=111, "Number Potentiometer Turns"=112, "Encoder Codes Per Rev"=113, "Pulse Width Decoded Position"=114, "Analog Position"=115, "Voltage Compensation Rate (V/s)"=116, "Slot 1 - Allowable Closed-Loop Error"=117, "Motion Profile Has Underrun Err"=119, "Reserved 120"=120, "Legacy Control Mode"=121, "Motion Magic Acceleration"=122, "Motion Magic Cruise Velocity"=123, "Status 10 Frame Rate"=124, "Current Limit Threshold"=125, "CustomParam0"=137, "CustomParam1"=138, "PersStorageSaving"=139, "ClearPositionOnLimitF"=144, "ClearPositionOnLimitR"=145, "NominalBatteryVoltage"=146, "SampleVelocityPeriod"=147, "SampleVelocityWindow"=148] ("Parameter")
          n64 = Unbundle By Name(w127) -> ("CAN.Device Number"=w128:u8)
          n65 = call <vilib>:"WPI_CANTalonSRX_SetParameter.vi"("Value"=0.0, "Parameter"=w129, "Device ID (0)"=w128) -> ()  [unwired: 7 in, 2 out]
        }
      }
    }
    frame "SHOOT" {
      n66 = call <vilib>:"WPI_CANTalonSRX_SetReference.vi"("error in (no error)"=w162, "Feedback Reference"=WPI_CANTalonSRX_APIFeedbackSelect."CTR Magnetic Enc (Relative)", "CAN Talon SRX Ref"=w163) -> ("error out"=w161:errorcluster, "CAN Talon SRX Ref"=w171:T7)  [unwired: 7 in]
      n67 = call <vilib>:"WPI_MotorControlSetOutput.vi"("error in (no error)"=w147, "Output"=0.75, "MotorControlDevRef"=w148) -> ("error out"=w144:errorcluster, "MotorControlDevRef"=w142:T7)  [unwired: 6 in, 1 out]
      n68 = call <vilib>:"WPI_CANTalonSRX_SetPID.vi"("CAN Talon SRX Ref"=w171, "P"=0.0, "I"=0.0, "D"=0.0, "error in (no error)"=w161, "F"=0.01, "I Zone"=0.0, "Ramp Rate"=0.0) -> ("CAN Talon SRX Ref"=w168:T7, "error out"=w160:errorcluster)  [unwired: 6 in]
      n69 = call <vilib>:"WPI_CANTalonSRX_ChangeMode.vi"("error in (no error)"=w160, "Output"=9800.0 ("y"), "Control Mode"=WPI_CANTalonSRX_APIControlMode."Speed", "CAN Talon SRX Ref"=w168) -> ("error out"=w159:errorcluster, "CAN Talon SRX Ref"=w164:T7)  [unwired: 6 in]
      n70 = call <vilib>:"WPI_CANTalonSRX_GetStatus.vi"("error in (no error)"=w159, "CAN Talon SRX Ref"=w164) -> ("error out"=w145:errorcluster)  [unwired: 7 in, 2 out]
      n71 = Merge Errors(w145, w144) -> (w143:errorcluster)
      n72 = call <vilib>:"WPI_RobotDriveDelayAndUpdateSafety.vi"("error in (no error)"=w143, "Delay (s)"=10.0, "RobotDriveDevRef"=w157) -> ("error out"=w141:errorcluster, "RobotDriveDevRef 2"=w158:T11)  [unwired: 7 in]
      n73 = call <vilib>:"WPI_MotorControlSetOutput.vi"("error in (no error)"=w141, "Output"=0.0, "MotorControlDevRef"=w142) -> ()  [unwired: 6 in, 3 out]
      n74 = call-poly <vilib>:"WPI_RobotDriveArcadeDrive.vi"("error in (no error)"=w141, "Y axis value"=0.0, "X axis value"=0.4, "RobotDriveDevRef"=w158) -> ("error out"=w154:errorcluster, "RobotDriveDevRef"=w155:T11)  [unwired: 5 in, 1 out]
      n75 = call <vilib>:"WPI_RobotDriveDelayAndUpdateSafety.vi"("error in (no error)"=w154, "Delay (s)"=1.0, "RobotDriveDevRef"=w155) -> ("error out"=w134:errorcluster, "RobotDriveDevRef 2"=w133:T11)  [unwired: 7 in]
      n76 = call-poly <vilib>:"WPI_RobotDriveArcadeDrive.vi"("error in (no error)"=w134, "Y axis value"=-0.6, "X axis value"=0.0, "RobotDriveDevRef"=w133) -> ("error out"=w137:errorcluster, "RobotDriveDevRef"=w138:T11)  [unwired: 5 in, 1 out]
      n77 = call <vilib>:"WPI_RobotDriveDelayAndUpdateSafety.vi"("error in (no error)"=w137, "Delay (s)"=3.0, "RobotDriveDevRef"=w138) -> ("error out"=w131:errorcluster, "RobotDriveDevRef 2"=w132:T11)  [unwired: 7 in]
      n78 = call-poly <vilib>:"WPI_RobotDriveArcadeDrive.vi"("error in (no error)"=w131, "Y axis value"=0.0, "X axis value"=0.0, "RobotDriveDevRef"=w132) -> ()  [unwired: 5 in, 3 out]
    }
    frame "SHOOTRED" {
      # "SHOOTRED"
      n79 = call <vilib>:"WPI_CANTalonSRX_SetReference.vi"("error in (no error)"=w228, "Feedback Reference"=WPI_CANTalonSRX_APIFeedbackSelect."CTR Magnetic Enc (Relative)", "CAN Talon SRX Ref"=w229) -> ("error out"=w227:errorcluster, "CAN Talon SRX Ref"=w237:T7)  [unwired: 7 in]
      n80 = call <vilib>:"WPI_MotorControlSetOutput.vi"("error in (no error)"=w215, "Output"=0.75, "MotorControlDevRef"=w216) -> ("error out"=w212:errorcluster, "MotorControlDevRef"=w210:T7)  [unwired: 6 in, 1 out]
      n81 = call <vilib>:"WPI_CANTalonSRX_SetPID.vi"("CAN Talon SRX Ref"=w237, "P"=0.0, "I"=0.0, "D"=0.0, "error in (no error)"=w227, "F"=0.01, "I Zone"=0.0, "Ramp Rate"=0.0) -> ("CAN Talon SRX Ref"=w234:T7, "error out"=w226:errorcluster)  [unwired: 6 in]
      n82 = call <vilib>:"WPI_CANTalonSRX_ChangeMode.vi"("error in (no error)"=w226, "Output"=9800.0 ("y"), "Control Mode"=WPI_CANTalonSRX_APIControlMode."Speed", "CAN Talon SRX Ref"=w234) -> ("error out"=w225:errorcluster, "CAN Talon SRX Ref"=w230:T7)  [unwired: 6 in]
      n83 = call <vilib>:"WPI_CANTalonSRX_GetStatus.vi"("error in (no error)"=w225, "CAN Talon SRX Ref"=w230) -> ("error out"=w213:errorcluster, "CAN Talon SRX Ref"=w195:T7)  [unwired: 7 in, 1 out]
      n84 = Merge Errors(w213, w212) -> (w211:errorcluster)
      n85 = call <vilib>:"WPI_RobotDriveDelayAndUpdateSafety.vi"("error in (no error)"=w211, "Delay (s)"=10.0, "RobotDriveDevRef"=w223) -> ("error out"=w194:errorcluster, "RobotDriveDevRef 2"=w224:T11)  [unwired: 7 in]
      n86 = call <vilib>:"WPI_CANTalonSRX_ChangeMode.vi"("error in (no error)"=w194, "Output"=0.0 ("y"), "Control Mode"=WPI_CANTalonSRX_APIControlMode."Speed", "CAN Talon SRX Ref"=w195) -> ("error out"=w196:errorcluster, "CAN Talon SRX Ref"=w197:T7)  [unwired: 6 in]
      n87 = call <vilib>:"WPI_MotorControlSetOutput.vi"("error in (no error)"=w194, "Output"=0.0, "MotorControlDevRef"=w210) -> ("error out"=w192:errorcluster)  [unwired: 6 in, 2 out]
      n88 = call <vilib>:"WPI_CANTalonSRX_GetStatus.vi"("error in (no error)"=w196, "CAN Talon SRX Ref"=w197) -> ("error out"=w193:errorcluster)  [unwired: 7 in, 2 out]
      n89 = Merge Errors(w193, w192) -> (w191:errorcluster)
      n90 = call <vilib>:"WPI_RobotDriveTankDrive.vi"("error in (no error)"=w191, "Right axis value"=0.6 ("Y axis value"), "Left axis value"=0.6, "RobotDriveDevRef"=w224) -> ("error out"=w221:errorcluster, "RobotDriveDevRef"=w222:T11)  [unwired: 5 in, 1 out]
      n91 = call <vilib>:"WPI_RobotDriveDelayAndUpdateSafety.vi"("error in (no error)"=w221, "Delay (s)"=0.25, "RobotDriveDevRef"=w222) -> ("error out"=w203:errorcluster, "RobotDriveDevRef 2"=w202:T11)  [unwired: 7 in]
      n92 = call-poly <vilib>:"WPI_RobotDriveArcadeDrive.vi"("error in (no error)"=w203, "Y axis value"=0.0, "X axis value"=-0.8, "RobotDriveDevRef"=w202) -> ("error out"=w206:errorcluster, "RobotDriveDevRef"=w207:T11)  [unwired: 5 in, 1 out]
      n93 = call <vilib>:"WPI_RobotDriveDelayAndUpdateSafety.vi"("error in (no error)"=w206, "Delay (s)"=0.5, "RobotDriveDevRef"=w207) -> ("error out"=w200:errorcluster, "RobotDriveDevRef 2"=w201:T11)  [unwired: 7 in]
      n94 = call-poly <vilib>:"WPI_RobotDriveArcadeDrive.vi"("error in (no error)"=w200, "Y axis value"=-0.5, "X axis value"=-0.55, "RobotDriveDevRef"=w201) -> ("error out"=w189:errorcluster, "RobotDriveDevRef"=w190:T11)  [unwired: 5 in, 1 out]
      n95 = call <vilib>:"WPI_RobotDriveDelayAndUpdateSafety.vi"("error in (no error)"=w189, "Delay (s)"=1.0, "RobotDriveDevRef"=w190) -> ("error out"=w187:errorcluster, "RobotDriveDevRef 2"=w186:T11)  [unwired: 7 in]
      n96 = call-poly <vilib>:"WPI_RobotDriveArcadeDrive.vi"("error in (no error)"=w187, "Y axis value"=-0.5 ("X axis value"), "RobotDriveDevRef"=w186) -> ("error out"=w181:errorcluster, "RobotDriveDevRef"=w182:T11)  [unwired: 6 in, 1 out]
      n97 = call <vilib>:"WPI_RobotDriveDelayAndUpdateSafety.vi"("error in (no error)"=w181, "Delay (s)"=2.0, "RobotDriveDevRef"=w182) -> ("error out"=w178:errorcluster, "RobotDriveDevRef 2"=w179:T11)  [unwired: 7 in]
      n98 = call-poly <vilib>:"WPI_RobotDriveArcadeDrive.vi"("error in (no error)"=w178, "Y axis value"=0.0, "X axis value"=0.0, "RobotDriveDevRef"=w179) -> ()  [unwired: 5 in, 3 out]
    }
    frame "NEW" {
      n99 = while {
        tunnel: w263 -> [w355]
        tunnel: w262 -> [w354]
        tunnel: [w348] -> w264
        tunnel: [w347] -> w265
        tunnel: w261 -> [w346]
        tunnel: w260 -> [w340]
        tunnel: [w336] -> w259
        tunnel: [w335] -> w258
        tunnel: w249 -> [w334]
        tunnel: [w334] -> w248
        stop <- w337 stop-if-true
        n100 = call <vilib>:"WPI_EncoderGet.vi"("EncoderDevRef"=w346) -> ("Distance"=w345:dbl, "EncoderDevRef"=w336:T3)  [unwired: 5 in, 4 out]
        n101 = call <vilib>:"WPI_EncoderGet.vi"("EncoderDevRef"=w355) -> ("Distance"=w353:dbl, "EncoderDevRef"=w347:T3)  [unwired: 5 in, 4 out]
        n102 = Greater?(x=w345, y=4.0) -> (0:w338:bool)
        n103 = Greater?(x=w353, y=4.0) -> (0:w339:bool)
        n104 = Select(t=0.0, s=w338, f=-0.3) -> (s? t:f=w341:dbl)
        n105 = Select(t=0.0, s=w339, f=-0.3) -> (s? t:f=w349:dbl)
        n106 = And(x=w339, y=w338) -> (x .and. y?=w337:bool)
        n107 = call <vilib>:"WPI_MotorControlSetOutput.vi"("Output"=w341, "MotorControlDevRef"=w340) -> ("MotorControlDevRef"=w335:T7)  [unwired: 7 in, 2 out]
        n108 = call <vilib>:"WPI_MotorControlSetOutput.vi"("Output"=w349, "MotorControlDevRef"=w354) -> ("MotorControlDevRef"=w348:T7)  [unwired: 7 in, 2 out]
      }
      n109 = while {
        tunnel: [w330] -> w257
        tunnel: [w329] -> w256
        tunnel: w265 -> [w328]
        tunnel: w264 -> [w327]
        tunnel: w259 -> [w323]
        tunnel: w258 -> [w322]
        tunnel: [w323] -> w255
        tunnel: [w322] -> w254
        tunnel: w248 -> [w321]
        tunnel: [w321] -> w247
        stop <- w324 continue-if-true
        n110 = call <vilib>:"WPI_EncoderGet.vi"("EncoderDevRef"=w328) -> ("Distance"=w326:dbl, "EncoderDevRef"=w330:T3)  [unwired: 5 in, 4 out]
        n111 = Greater?(x=4.0 ("y"), y=w326) -> (0:w324:bool)
        n112 = Select(t=0.3, s=w324, f=0.0 ("Output")) -> (s? t:f=w331:dbl)
        n113 = call <vilib>:"WPI_MotorControlSetOutput.vi"("Output"=w331, "MotorControlDevRef"=w327) -> ("MotorControlDevRef"=w329:T7)  [unwired: 7 in, 2 out]
      }
      n114 = while {
        tunnel: w257 -> [w320]
        tunnel: w256 -> [w319]
        tunnel: [w313] -> w250
        tunnel: [w312] -> w251
        tunnel: w255 -> [w311]
        tunnel: w254 -> [w305]
        tunnel: [w301] -> w252
        tunnel: [w300] -> w253
        tunnel: w247 -> [w299]
        tunnel: [w299] -> w246
        stop <- w302 stop-if-true
        n115 = call <vilib>:"WPI_EncoderGet.vi"("EncoderDevRef"=w311) -> ("Distance"=w310:dbl, "EncoderDevRef"=w301:T3)  [unwired: 5 in, 4 out]
        n116 = call <vilib>:"WPI_EncoderGet.vi"("EncoderDevRef"=w320) -> ("Distance"=w318:dbl, "EncoderDevRef"=w312:T3)  [unwired: 5 in, 4 out]
        n117 = Greater?(x=w310, y=4.0) -> (0:w303:bool)
        n118 = Greater?(x=w318, y=4.0) -> (0:w304:bool)
        n119 = Select(t=0.0, s=w303, f=-0.3) -> (s? t:f=w306:dbl)
        n120 = Select(t=0.0, s=w304, f=-0.3) -> (s? t:f=w314:dbl)
        n121 = And(x=w304, y=w303) -> (x .and. y?=w302:bool)
        n122 = call <vilib>:"WPI_MotorControlSetOutput.vi"("Output"=w306, "MotorControlDevRef"=w305) -> ("MotorControlDevRef"=w300:T7)  [unwired: 7 in, 2 out]
        n123 = call <vilib>:"WPI_MotorControlSetOutput.vi"("Output"=w314, "MotorControlDevRef"=w319) -> ("MotorControlDevRef"=w313:T7)  [unwired: 7 in, 2 out]
      }
      n124 = while {
        tunnel: w253 -> [w290]
        tunnel: w252 -> [w289]
        tunnel: w251 -> [w287]
        tunnel: w250 -> [w288]
        tunnel: w246 -> [w298]
        tunnel: [w290] -> w245
        tunnel: [w289] -> w244
        tunnel: [w288] -> w243
        tunnel: [w287] -> w242
        stop <- w291 stop-if-true
        n125 = global read "Robot Global Data.vi" "LOWER LIMIT"() -> (w294:bool)
        n126 = Select(t=0.0, s=w294, f=-0.5) -> (s? t:f=w295:dbl)
        n127 = call <vilib>:"WPI_MotorControlSetOutput.vi"("Output"=w295, "MotorControlDevRef"=w298) -> ("Motor Output"=w293:dbl)  [unwired: 7 in, 2 out]
        n128 = Equal?(x=w293, y=0.0) -> (x = y?=w291:bool)
      }
      n129 = while {
        tunnel: [w281] -> _
        tunnel: [w280] -> _
        tunnel: [w271] -> _
        tunnel: [w270] -> _
        tunnel: w245 -> [w269]
        tunnel: w244 -> [w268]
        tunnel: w243 -> [w267]
        tunnel: w242 -> [w266]
        stop <- w272 stop-if-true
        n130 = call <vilib>:"WPI_EncoderGet.vi"("EncoderDevRef"=w268) -> ("Distance"=w279:dbl, "EncoderDevRef"=w271:T3)  [unwired: 5 in, 4 out]
        n131 = call <vilib>:"WPI_EncoderGet.vi"("EncoderDevRef"=w266) -> ("Distance"=w286:dbl, "EncoderDevRef"=w280:T3)  [unwired: 5 in, 4 out]
        n132 = Greater?(x=w279, y=0.0) -> (0:w273:bool)
        n133 = Greater?(x=w286, y=0.0) -> (0:w274:bool)
        n134 = Select(t=-0.3, s=w273, f=0.0) -> (s? t:f=w275:dbl)
        n135 = Select(t=-0.3, s=w274, f=0.0) -> (s? t:f=w282:dbl)
        n136 = And(x=w274, y=w273) -> (x .and. y?=w272:bool)
        n137 = call <vilib>:"WPI_MotorControlSetOutput.vi"("Output"=w275, "MotorControlDevRef"=w269) -> ("MotorControlDevRef"=w270:T7)  [unwired: 7 in, 2 out]
        n138 = call <vilib>:"WPI_MotorControlSetOutput.vi"("Output"=w282, "MotorControlDevRef"=w267) -> ("MotorControlDevRef"=w281:T7)  [unwired: 7 in, 2 out]
      }
    }
    frame "MIDDLE" {
      n139 = call-poly <vilib>:"WPI_RobotDriveArcadeDrive.vi"("error in (no error)"=w385, "Y axis value"=0.45, "RobotDriveDevRef"=w386) -> ("error out"=w382:errorcluster, "RobotDriveDevRef"=w383:T11)  [unwired: 6 in, 1 out]
      n140 = call <vilib>:"WPI_RobotDriveDelayAndUpdateSafety.vi"("error in (no error)"=w382, "Delay (s)"=2.0, "RobotDriveDevRef"=w383) -> ("error out"=w380:errorcluster, "RobotDriveDevRef 2"=w379:T11)  [unwired: 7 in]
      n141 = call-poly <vilib>:"WPI_RobotDriveArcadeDrive.vi"("error in (no error)"=w380, "Y axis value"=0.0, "RobotDriveDevRef"=w379) -> ("error out"=w376:errorcluster, "RobotDriveDevRef"=w377:T11)  [unwired: 6 in, 1 out]
      n142 = call <vilib>:"WPI_RobotDriveDelayAndUpdateSafety.vi"("error in (no error)"=w376, "Delay (s)"=0.5, "RobotDriveDevRef"=w377) -> ("error out"=w374:errorcluster, "RobotDriveDevRef 2"=w372:T11)  [unwired: 7 in]
      n143 = call <vilib>:"WPI_MotorControlSetOutput.vi"("error in (no error)"=w374, "Output"=-0.7, "MotorControlDevRef"=w373) -> ("error out"=w371:errorcluster, "MotorControlDevRef"=w367:T7)  [unwired: 6 in, 1 out]
      n144 = call <vilib>:"WPI_RobotDriveDelayAndUpdateSafety.vi"("error in (no error)"=w371, "Delay (s)"=1.5, "RobotDriveDevRef"=w372) -> ("error out"=w368:errorcluster, "RobotDriveDevRef 2"=w365:T11)  [unwired: 7 in]
      n145 = call <vilib>:"WPI_MotorControlSetOutput.vi"("error in (no error)"=w368, "Output"=0.0, "MotorControlDevRef"=w367) -> ("error out"=w364:errorcluster)  [unwired: 6 in, 2 out]
      n146 = call-poly <vilib>:"WPI_RobotDriveArcadeDrive.vi"("error in (no error)"=w364, "Y axis value"=-0.4, "RobotDriveDevRef"=w365) -> ("error out"=w361:errorcluster, "RobotDriveDevRef"=w362:T11)  [unwired: 6 in, 1 out]
      n147 = call <vilib>:"WPI_RobotDriveDelayAndUpdateSafety.vi"("error in (no error)"=w361, "Delay (s)"=2.0, "RobotDriveDevRef"=w362) -> ("error out"=w358:errorcluster, "RobotDriveDevRef 2"=w359:T11)  [unwired: 7 in]
      n148 = call-poly <vilib>:"WPI_RobotDriveArcadeDrive.vi"("error in (no error)"=w358, "Y axis value"=0.0, "X axis value"=0.0, "RobotDriveDevRef"=w359) -> ()  [unwired: 5 in, 3 out]
    }
    frame "RIGHTSIDE" {
      # "RIGHTSIDE"
      n149 = call-poly <vilib>:"WPI_RobotDriveArcadeDrive.vi"("error in (no error)"=w388, "Y axis value"=0.59, "RobotDriveDevRef"=w389) -> ("error out"=w428:errorcluster, "RobotDriveDevRef"=w429:T11)  [unwired: 6 in, 1 out]
      n150 = call <vilib>:"WPI_RobotDriveDelayAndUpdateSafety.vi"("error in (no error)"=w428, "Delay (s)"=1.8, "RobotDriveDevRef"=w429) -> ("error out"=w424:errorcluster, "RobotDriveDevRef 2"=w425:T11)  [unwired: 7 in]
      n151 = call-poly <vilib>:"WPI_RobotDriveArcadeDrive.vi"("error in (no error)"=w424, "X axis value"=0.36, "RobotDriveDevRef"=w425) -> ("error out"=w421:errorcluster, "RobotDriveDevRef"=w422:T11)  [unwired: 6 in, 1 out]
      n152 = call <vilib>:"WPI_RobotDriveDelayAndUpdateSafety.vi"("error in (no error)"=w421, "Delay (s)"=1.0, "RobotDriveDevRef"=w422) -> ("error out"=w418:errorcluster, "RobotDriveDevRef 2"=w419:T11)  [unwired: 7 in]
      n153 = call-poly <vilib>:"WPI_RobotDriveArcadeDrive.vi"("error in (no error)"=w418, "Y axis value"=0.5, "RobotDriveDevRef"=w419) -> ("error out"=w415:errorcluster, "RobotDriveDevRef"=w416:T11)  [unwired: 6 in, 1 out]
      n154 = call <vilib>:"WPI_RobotDriveDelayAndUpdateSafety.vi"("error in (no error)"=w415, "Delay (s)"=2.3, "RobotDriveDevRef"=w416) -> ("error out"=w412:errorcluster, "RobotDriveDevRef 2"=w413:T11)  [unwired: 7 in]
      n155 = call-poly <vilib>:"WPI_RobotDriveArcadeDrive.vi"("error in (no error)"=w412, "Y axis value"=0.0, "RobotDriveDevRef"=w413) -> ("error out"=w409:errorcluster, "RobotDriveDevRef"=w410:T11)  [unwired: 6 in, 1 out]
      n156 = call <vilib>:"WPI_RobotDriveDelayAndUpdateSafety.vi"("error in (no error)"=w409, "Delay (s)"=0.5, "RobotDriveDevRef"=w410) -> ("error out"=w407:errorcluster, "RobotDriveDevRef 2"=w405:T11)  [unwired: 7 in]
      n157 = call <vilib>:"WPI_MotorControlSetOutput.vi"("error in (no error)"=w407, "Output"=-0.7, "MotorControlDevRef"=w387) -> ("error out"=w404:errorcluster, "MotorControlDevRef"=w393:T7)  [unwired: 6 in, 1 out]
      n158 = call <vilib>:"WPI_RobotDriveDelayAndUpdateSafety.vi"("error in (no error)"=w404, "Delay (s)"=1.5, "RobotDriveDevRef"=w405) -> ("error out"=w392:errorcluster, "RobotDriveDevRef 2"=w402:T11)  [unwired: 7 in]
      n159 = call <vilib>:"WPI_MotorControlSetOutput.vi"("error in (no error)"=w392, "Output"=0.0, "MotorControlDevRef"=w393) -> ("error out"=w390:errorcluster)  [unwired: 6 in, 2 out]
      n160 = call-poly <vilib>:"WPI_RobotDriveArcadeDrive.vi"("error in (no error)"=w390, "Y axis value"=-0.4, "RobotDriveDevRef"=w402) -> ("error out"=w399:errorcluster, "RobotDriveDevRef"=w400:T11)  [unwired: 6 in, 1 out]
      n161 = call <vilib>:"WPI_RobotDriveDelayAndUpdateSafety.vi"("error in (no error)"=w399, "Delay (s)"=2.0, "RobotDriveDevRef"=w400) -> ("error out"=w397:errorcluster, "RobotDriveDevRef 2"=w396:T11)  [unwired: 7 in]
      n162 = call-poly <vilib>:"WPI_RobotDriveArcadeDrive.vi"("error in (no error)"=w397, "Y axis value"=0.0, "X axis value"=0.0, "RobotDriveDevRef"=w396) -> ()  [unwired: 5 in, 3 out]
    }
    frame "LEFTSIDE" {
      n163 = call-poly <vilib>:"WPI_RobotDriveArcadeDrive.vi"("error in (no error)"=w471, "Y axis value"=0.6, "RobotDriveDevRef"=w472) -> ("error out"=w469:errorcluster, "RobotDriveDevRef"=w470:T11)  [unwired: 6 in, 1 out]
      n164 = call <vilib>:"WPI_RobotDriveDelayAndUpdateSafety.vi"("error in (no error)"=w469, "Delay (s)"=2.0, "RobotDriveDevRef"=w470) -> ("error out"=w465:errorcluster, "RobotDriveDevRef 2"=w466:T11)  [unwired: 7 in]
      n165 = call-poly <vilib>:"WPI_RobotDriveArcadeDrive.vi"("error in (no error)"=w465, "X axis value"=-0.45, "RobotDriveDevRef"=w466) -> ("error out"=w462:errorcluster, "RobotDriveDevRef"=w463:T11)  [unwired: 6 in, 1 out]
      n166 = call <vilib>:"WPI_RobotDriveDelayAndUpdateSafety.vi"("error in (no error)"=w462, "Delay (s)"=1.0, "RobotDriveDevRef"=w463) -> ("error out"=w459:errorcluster, "RobotDriveDevRef 2"=w460:T11)  [unwired: 7 in]
      n167 = call-poly <vilib>:"WPI_RobotDriveArcadeDrive.vi"("error in (no error)"=w459, "Y axis value"=0.52, "RobotDriveDevRef"=w460) -> ("error out"=w456:errorcluster, "RobotDriveDevRef"=w457:T11)  [unwired: 6 in, 1 out]
      n168 = call <vilib>:"WPI_RobotDriveDelayAndUpdateSafety.vi"("error in (no error)"=w456, "Delay (s)"=2.25, "RobotDriveDevRef"=w457) -> ("error out"=w453:errorcluster, "RobotDriveDevRef 2"=w454:T11)  [unwired: 7 in]
      n169 = call-poly <vilib>:"WPI_RobotDriveArcadeDrive.vi"("error in (no error)"=w453, "Y axis value"=0.0, "RobotDriveDevRef"=w454) -> ("error out"=w450:errorcluster, "RobotDriveDevRef"=w451:T11)  [unwired: 6 in, 1 out]
      n170 = call <vilib>:"WPI_RobotDriveDelayAndUpdateSafety.vi"("error in (no error)"=w450, "Delay (s)"=0.5, "RobotDriveDevRef"=w451) -> ("error out"=w447:errorcluster, "RobotDriveDevRef 2"=w445:T11)  [unwired: 7 in]
      n171 = call <vilib>:"WPI_MotorControlSetOutput.vi"("error in (no error)"=w447, "Output"=-0.7, "MotorControlDevRef"=w448) -> ("error out"=w444:errorcluster, "MotorControlDevRef"=w433:T7)  [unwired: 6 in, 1 out]
      n172 = call <vilib>:"WPI_RobotDriveDelayAndUpdateSafety.vi"("error in (no error)"=w444, "Delay (s)"=1.5, "RobotDriveDevRef"=w445) -> ("error out"=w432:errorcluster, "RobotDriveDevRef 2"=w442:T11)  [unwired: 7 in]
      n173 = call <vilib>:"WPI_MotorControlSetOutput.vi"("error in (no error)"=w432, "Output"=0.0, "MotorControlDevRef"=w433) -> ("error out"=w430:errorcluster)  [unwired: 6 in, 2 out]
      n174 = call-poly <vilib>:"WPI_RobotDriveArcadeDrive.vi"("error in (no error)"=w430, "Y axis value"=-0.4, "RobotDriveDevRef"=w442) -> ("error out"=w439:errorcluster, "RobotDriveDevRef"=w440:T11)  [unwired: 6 in, 1 out]
      n175 = call <vilib>:"WPI_RobotDriveDelayAndUpdateSafety.vi"("error in (no error)"=w439, "Delay (s)"=2.0, "RobotDriveDevRef"=w440) -> ("error out"=w437:errorcluster, "RobotDriveDevRef 2"=w436:T11)  [unwired: 7 in]
      n176 = call-poly <vilib>:"WPI_RobotDriveArcadeDrive.vi"("error in (no error)"=w437, "Y axis value"=0.0, "X axis value"=0.0, "RobotDriveDevRef"=w436) -> ()  [unwired: 5 in, 3 out]
    }
    frame "Forward" {
      n177 = call-poly <vilib>:"WPI_RobotDriveArcadeDrive.vi"("error in (no error)"=w477, "Y axis value"=0.55, "RobotDriveDevRef"=w478) -> ("error out"=w473:errorcluster, "RobotDriveDevRef"=w475:T11)  [unwired: 6 in, 1 out]
      n178 = call <vilib>:"WPI_RobotDriveDelayAndUpdateSafety.vi"("error in (no error)"=w473, "Delay (s)"=2.8, "RobotDriveDevRef"=w475) -> ()  [unwired: 7 in, 2 out]
    }
    frame "GEAR DROP" {
      n179 = call-poly <vilib>:"WPI_RobotDriveArcadeDrive.vi"("error in (no error)"=w502, "Y axis value"=0.45, "RobotDriveDevRef"=w503) -> ("error out"=w499:errorcluster, "RobotDriveDevRef"=w500:T11)  [unwired: 6 in, 1 out]
      n180 = call <vilib>:"WPI_RobotDriveDelayAndUpdateSafety.vi"("error in (no error)"=w499, "Delay (s)"=2.4, "RobotDriveDevRef"=w500) -> ("error out"=w497:errorcluster, "RobotDriveDevRef 2"=w496:T11)  [unwired: 7 in]
      n181 = call-poly <vilib>:"WPI_RobotDriveArcadeDrive.vi"("error in (no error)"=w497, "Y axis value"=0.0, "RobotDriveDevRef"=w496) -> ("error out"=w493:errorcluster, "RobotDriveDevRef"=w494:T11)  [unwired: 6 in, 1 out]
      n182 = call <vilib>:"WPI_RobotDriveDelayAndUpdateSafety.vi"("error in (no error)"=w493, "Delay (s)"=0.5, "RobotDriveDevRef"=w494) -> ("error out"=w486:errorcluster, "RobotDriveDevRef 2"=w485:T11)  [unwired: 7 in]
      n183 = while {
        tunnel: w486 -> [w515]
        tunnel: [w512] -> w484
        tunnel: w483 -> [w511]
        tunnel: [w510] -> w482
        stop <- w513 stop-if-true
        n184 = global read "Robot Global Data.vi" "LOWER LIMIT"() -> (w513:bool)
        n185 = call <vilib>:"WPI_MotorControlSetOutput.vi"("error in (no error)"=w515, "Output"=-0.6 ("f"), "MotorControlDevRef"=w511) -> ("error out"=w512:errorcluster, "MotorControlDevRef"=w510:T7)  [unwired: 6 in, 1 out]
      }
      n186 = call-poly <vilib>:"WPI_RobotDriveArcadeDrive.vi"("error in (no error)"=w484, "Y axis value"=-0.4, "RobotDriveDevRef"=w485) -> ("error out"=w490:errorcluster, "RobotDriveDevRef"=w489:T11)  [unwired: 6 in, 1 out]
      n187 = call <vilib>:"WPI_RobotDriveDelayAndUpdateSafety.vi"("error in (no error)"=w490, "Delay (s)"=1.5, "RobotDriveDevRef"=w489) -> ("error out"=w481:errorcluster)  [unwired: 7 in, 1 out]
      n188 = while {
        tunnel: w482 -> [w508]
        tunnel: w481 -> [w506]
        tunnel: [w505] -> w480
        tunnel: [w504] -> w479
        stop <- w509 stop-if-true
        n189 = call <vilib>:"WPI_MotorControlSetOutput.vi"("error in (no error)"=w506, "Output"=0.6, "MotorControlDevRef"=w508) -> ("error out"=w504:errorcluster, "MotorControlDevRef"=w505:T7)  [unwired: 6 in, 1 out]
        n190 = global read "Robot Global Data.vi" "UPPER LIMIT"() -> (w509:bool)
      }
      n191 = call <vilib>:"WPI_MotorControlSetOutput.vi"("error in (no error)"=w479, "Output"=0.0, "MotorControlDevRef"=w480) -> ()  [unwired: 6 in, 3 out]
    }
  }
